vi "Test Matrix Transpose.vi"() -> ()   [LabVIEW 2014, in "Arduino MatrixMath.lvlib"]
uses:
  Arduino MatrixMath.lvlib
panel:
  out "transposed A":sgl[](array[numeric])
  in  "A":sgl[](array[numeric])
  out "Error Out":errorcluster
  in  "Error In":errorcluster
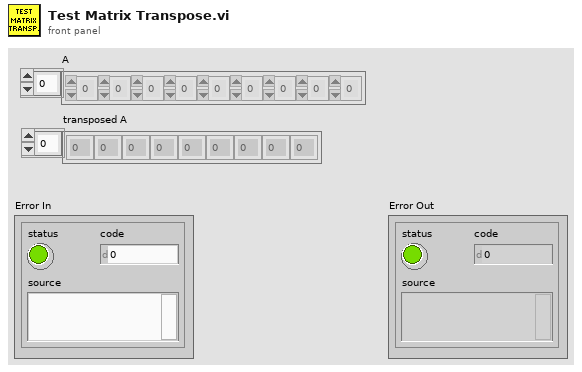
[diagram p1: front panel]
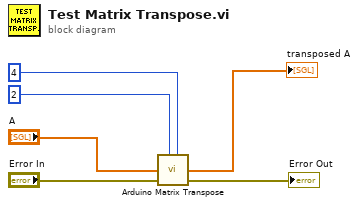
[diagram p0: block diagram]
diagram:
  n1 = call "Arduino Matrix Transpose.vi"("rows num."=u8 2, "A"="A", "Error In"="Error In", "cols num."=u8 4) -> ("transposed A"=→"transposed A":sgl[], "Error Out"=→"Error Out":errorcluster)  [unwired: 4 in]
